vi "READSTAT.vi"(0 "SPI Config In":T1) -> (1 "SPI Config Out":T1, 2 "Frames Read":u8[](array[numeric]) format="%b")   [LabVIEW 2019]
uses:
  SPI/SPI Config.ctl
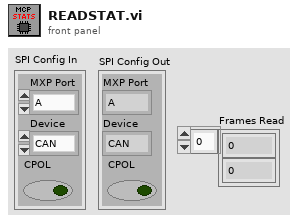
[diagram p1: front panel]
types:
  T1 = typedef "SPI Config.ctl" = cluster{"MXP Port":enum16{"A", "B"}, "Device":enum16{"CAN", "ENC", "IMU1", "IMU2"}, "CPOL":bool}
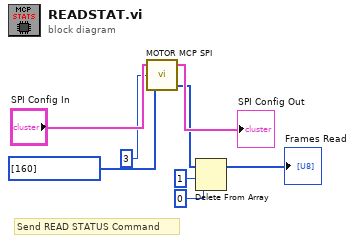
[diagram p0: block diagram]
diagram:
  # "Send READ STATUS Command"
  n1 = call "MOTOR MCP SPI.vi"("Data to Write"=u8[] [160] ("Frames to Write"), "Frames to Write"=u8 3, "SPI Config In"="SPI Config In") -> ("Data Read"=w1:u8[], "SPI Config Out"=→"SPI Config Out":T1)  [unwired: 1 out]
  n2 = Delete From Array(array=w1, length=1, index=0) -> (array with subset deleted=→"Frames Read":u8[])  [unwired: 1 out]
